vi "Test System.vi"() -> ()   [LabVIEW 2016]
panel:
  out "Velocity\n 2":dbl
  in  "Accel":dbl
  out "Velocity":dbl
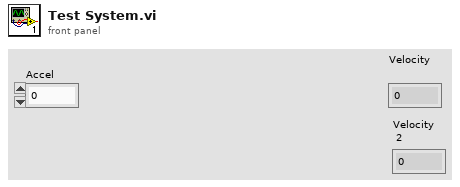
[diagram p1: front panel]
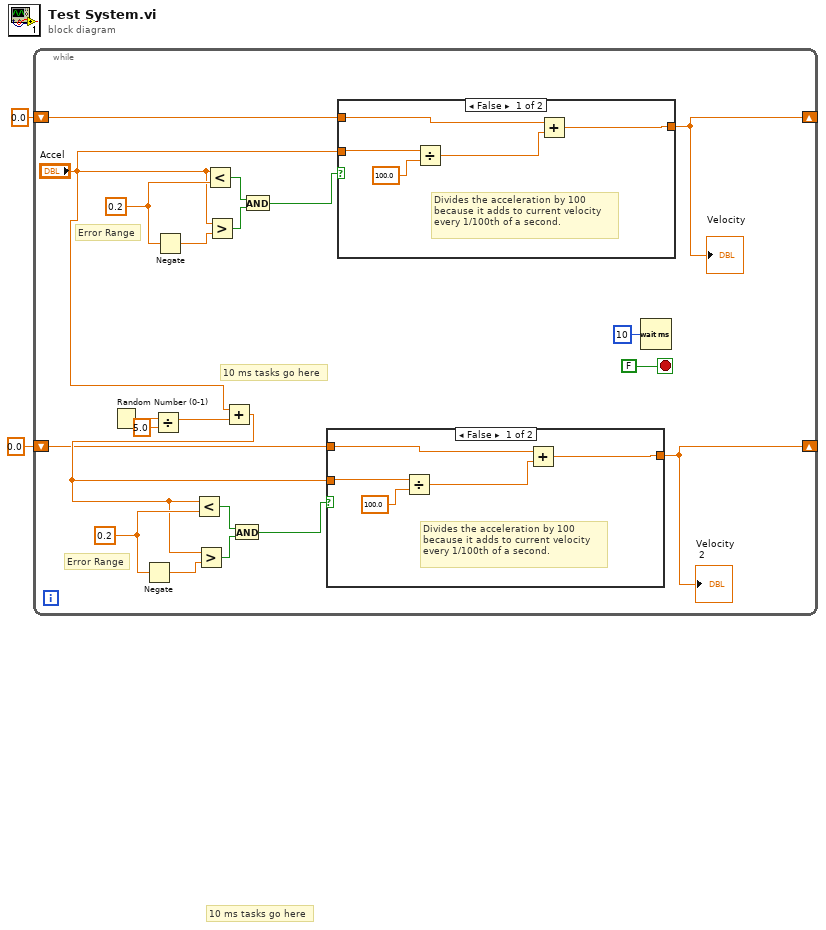
[diagram p0: block diagram]
diagram:
  # "10 ms tasks go here"
  n1 = while {
    shift-right: [w16] -> _
    shift-left: 0.0 -> [w15]
    shift-right: [w4] -> _
    shift-left: 0.0 -> [w3]
    stop <- FALSE stop-if-true
    w9 = 0.2 ("y")
    w20 = 0.2 ("y")
    # "Error Range"
    # "10 ms tasks go here"
    # "Error Range"
    n2 = Random Number (0-1)() -> (number: 0 to 1=w13:dbl)
    n3 = Negate(x=w9) -> (-x=w8:dbl)
    n4 = Divide(x=w13, y=5.0) -> (x/y=w6:dbl)
    n5 = Negate(x=w20) -> (-x=w21:dbl)
    n6 = Less?(x="Accel", y=w20) -> (x < y?=w19:bool)
    n7 = Greater?(x="Accel", y=w21) -> (0:w18:bool)
    n8 = Add(x="Accel", y=w6) -> (x+y=w5:dbl)
    n9 = Less?(x=w5, y=w9) -> (x < y?=w10:bool)
    n10 = Greater?(x=w5, y=w8) -> (0:w11:bool)
    n11 = And(x=w10, y=w11) -> (x .and. y?=w12:bool)
    n12 = And(x=w19, y=w18) -> (x .and. y?=w17:bool)
    n13 = case shown="False" w12 {
      tunnel: w5 -> [w26 _]
      tunnel: [w27 w29] -> w4
      tunnel: w3 -> [w28 w29]
      frame False {
        # "Divides the acceleration by 100\nbecause it adds to current velocity \nevery 1/100th of a second."
        n14 = Divide(x=w26, y=100.0) -> (x/y=w25:dbl)
        n15 = Add(x=w28, y=w25) -> (x+y=w27:dbl)
      }
      frame True {
      }
    }
    "Velocity\n 2" <- w4
    n16 = case shown="False" w17 {
      tunnel: "Accel" -> [w32 _]
      tunnel: [w33 w35] -> w16
      tunnel: w15 -> [w34 w35]
      frame False {
        # "Divides the acceleration by 100\nbecause it adds to current velocity \nevery 1/100th of a second."
        n17 = Divide(x=w32, y=100.0) -> (x/y=w31:dbl)
        n18 = Add(x=w34, y=w31) -> (x+y=w33:dbl)
      }
      frame True {
      }
    }
    "Velocity" <- w16
    n19 = Wait (ms)(milliseconds to wait=u32 10) -> ()  [unwired: 1 out]
  }
